vi "Plugin - Random Data Chart.vi"() -> ()   [LabVIEW 2016]
doc: "乱数値とユーザ指定値の積を波形チャートに表示するサブパネルプラグインVI。"
panel:
  in  "乗数":dbl(slide)=2.0 scale=0.0..10.0
  in  "パラメータ":string[](array[string])
  out "乱数チャート":dbl(graph)
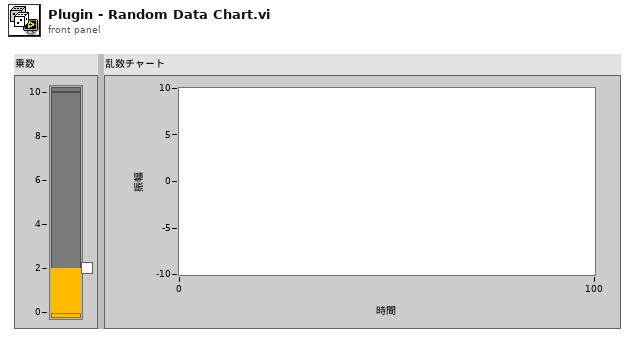
[diagram p1: front panel]
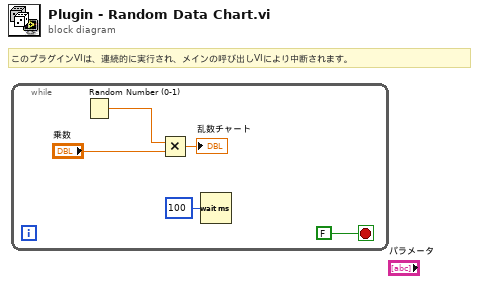
[diagram p0: block diagram]
diagram:
  # "このプラグインVIは、連続的に実行され、メインの呼び出しVIにより中断されます。"
  n1 = while {
    stop <- FALSE stop-if-true
    n2 = Random Number (0-1)() -> (number: 0 to 1=w2:dbl)
    n3 = Multiply(x=w2, y="乗数") -> (x*y=→"乱数チャート":dbl)
    n4 = Wait (ms)(milliseconds to wait=u32 100) -> ()  [unwired: 1 out]
  }
